vi "Mean_fr_NaN_data.vi"(0 "Data":dbl[](array[numeric]) format="%.2f") -> (1 "Mean value":dbl format="%.2f", 2 "GoodFraction":dbl)   [LabVIEW 2012]
uses:
  <vilib>/Analysis/baseanly.llb/Mean (DBL).vi
  <vilib>/Analysis/NI_AALBase.lvlib
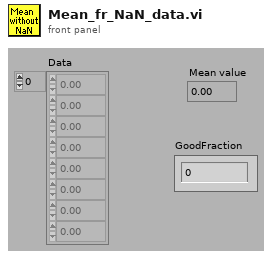
[diagram p1: front panel]
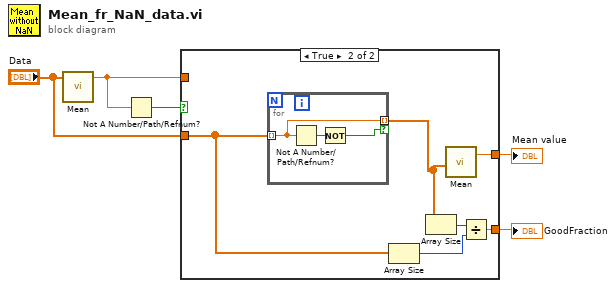
[diagram p0: block diagram]
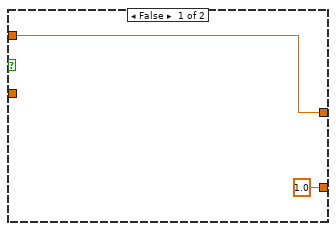
[diagram p2: hidden frame]
diagram:
  n1 = call-poly <vilib>:"Mean.vi"("X"="Data") -> ("mean"=w3:dbl)  [unwired: 1 out]
  n2 = Not A Number/Path/Refnum?(number/path/refnum=w3) -> (NaN/Path/Refnum?=w2:bool)
  n3 = case shown="True" w2 {
    tunnel: "Data" -> [_ w12]
    tunnel: [w7 w13] -> w4
    tunnel: w3 -> [w7 _]
    tunnel: [1.0 w9] -> w1
    frame False {
    }
    frame True {
      n4 = for {
        tunnel: w12 -> [w15] mode=indexing
        tunnel: [w15] -> w8 mode=indexing if=w14
        n5 = Not A Number/Path/Refnum?(number/path/refnum=w15) -> (NaN/Path/Refnum?=w16:bool)
        n6 = Not(x=w16) -> (.not. x?=w14:bool)
      }
      n7 = Array Size(array=w12) -> (size(s)=w10:i32)
      n8 = Array Size(array=w8) -> (size(s)=w11:i32)
      n9 = call-poly <vilib>:"Mean.vi"("X"=w8) -> ("mean"=w13:dbl)  [unwired: 1 out]
      n10 = Divide(x=w11, y=w10) -> (x/y=w9:dbl)
    }
  }
  "Mean value" <- w4
  "GoodFraction" <- w1
